vi "PRIME Detector Process File.vi"(8 "error in (no error)":errorcluster, 9 "Frame":i32, 10 "Camera":i32, 11 "Filename":string) -> (0 "error out":errorcluster, 2 "Keep?":bool, 3 "Image Data":T1)   [LabVIEW 2024]
uses:
  Detector Image typedef cluster.ctl
  Detector Class.lvclass
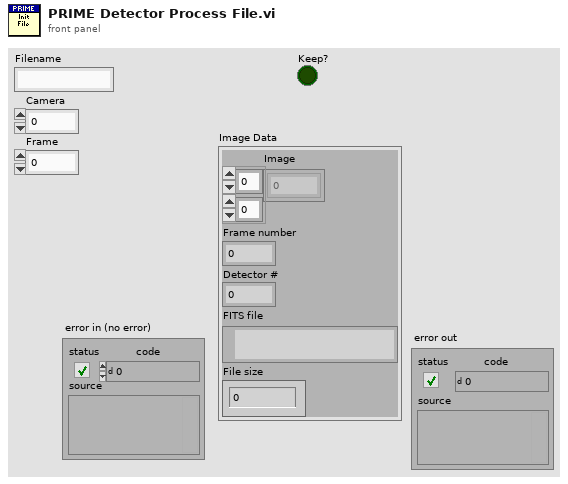
[diagram p1: front panel]
types:
  T1 = typedef "Detector Class.lvclass/Detector Image typedef cluster.ctl" = cluster{"Image":sgl[][], "Frame number":i32, "Detector #":u16, "FITS file":path, "File size":i64}
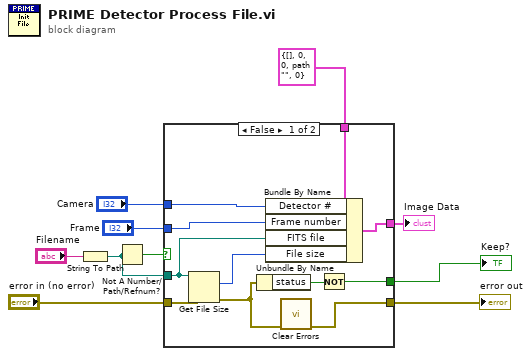
[diagram p0: block diagram]
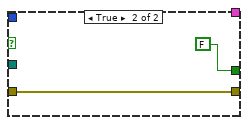
[diagram p2: hidden frame]
diagram:
  n1 = String To Path(string="Filename") -> (path=w10:path)
  n2 = Not A Number/Path/Refnum?(number/path/refnum=w10) -> (NaN/Path/Refnum?=w9:bool)
  n3 = case shown="False" w9 {
    tunnel: T1 {"Image"=[], "Frame number"=0, "Detector #"=0, "FITS file"=path "", "File size"=0} ("Image Data") -> [w21 _]
    tunnel: "Frame" -> [w20 _]
    tunnel: "Camera" -> [w19 _]
    tunnel: [w18 _] -> w1
    tunnel: w10 -> [w11 _]
    tunnel: [w15 FALSE] -> w2
    tunnel: "error in (no error)" -> [w14 w22]
    tunnel: [w13 w22] -> w3
    frame False {
      n4 = Get File Size(file=w11, error in=w14) -> (size (in bytes)=w12:i64, 0:w17:errorcluster)  [unwired: 1 out]
      n5 = Unbundle By Name(w17) -> ("status"=w16:bool)
      n6 = Bundle By Name(cluster=w21, "Detector #"=w19, "Frame number"=w20, "FITS file"=w11, "File size"=w12) -> (w18:T1)
      n7 = call <vilib>:"Clear Errors.vi"("error in (no error)"=w17) -> ("error out"=w13:errorcluster)  [unwired: 5 in, 1 out]
      n8 = Not(x=w16) -> (.not. x?=w15:bool)
    }
    frame True {
    }
  }
  "error out" <- w3
  "Keep?" <- w2
  "Image Data" <- w1
